vi "Create Sequence Call Step.vi"(8 "error in (no error)":errorcluster, 11 "QPA Measurement in":refnum<class "QPA Measurement.lvclass">) -> (0 "error out":errorcluster, 2 "Step Reference":refnum<k7>, 3 "QPA Measurement out":refnum<class "QPA Measurement.lvclass">)   [LabVIEW 2016, in "QPA Measurement.lvlib" / "QPA Measurement.lvclass"]
uses:
  QPA Measurement.lvclass
  C:/Projects/STS/Common/Sequence Automation/Plugins/Measurement Interface.lvlibp/Measurement Interface.lvclass
  QPA Measurement.lvclass/QPA Measurement.ctl
  Protected Methods/Read Sequence Reference.vi
  Protected Methods/Read Measurement Name.vi
  Plugins/Measurement Interface.lvlibp/Private Methods/Engine Reference/Read Engine Reference.vi
  Plugins/Measurement Interface.lvlibp/Private Methods/Measurement Parameters/Read Measurement Parameters.vi
  Plugins/String Database.lvlibp/String Database.lvclass
  Plugins/TestStand API Tools (TSAT).lvlibp/Step Actions/TSAT Step Actions.lvlib
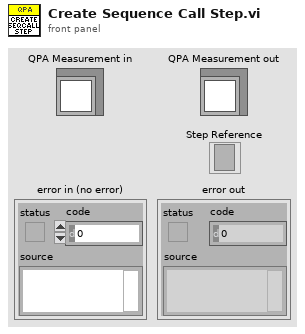
[diagram p1: front panel]
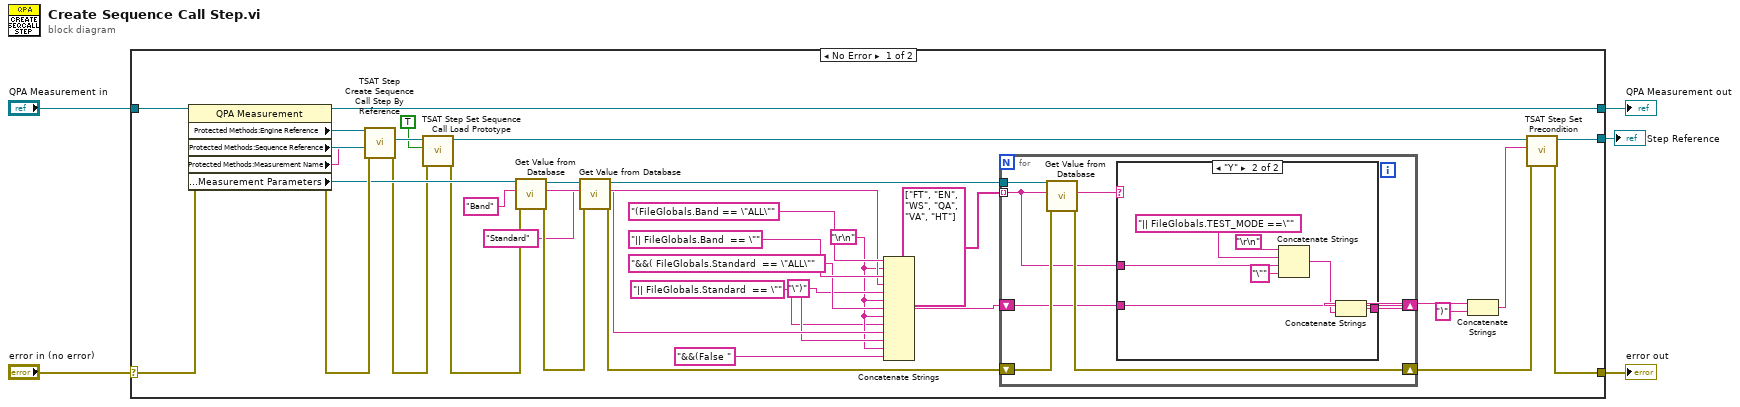
[diagram p0: block diagram]
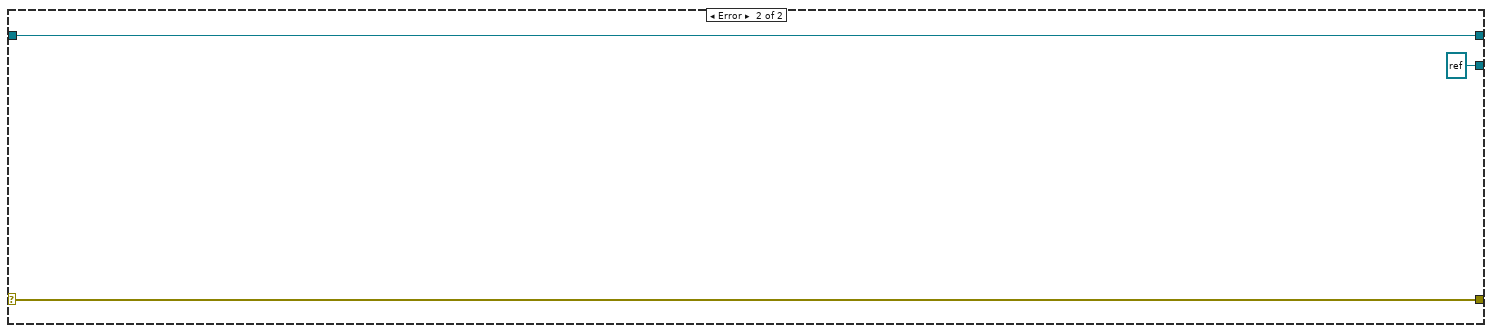
[diagram p3: hidden frame]
diagram:
  n1 = case shown="No Error" "error in (no error)" {
    selector: "error in (no error)" -> [w41 w59]
    tunnel: [w30 w59] -> w4
    tunnel: [w39 w58] -> w2
    tunnel: "QPA Measurement in" -> [w40 w58]
    tunnel: [w34 refnum<k7> refnum ("Step Reference")] -> w1
    frame No Error {
      w7 = "\r\n"
      w8 = "\")" ("string")
      n2 = property class="QPA Measurement"(reference=w40, error in=w41) -> (reference out=w39:refnum<class "QPA Measurement.lvclass">, error out=w35:errorcluster, "Protected Methods:Engine Reference"=w38:refnum<k7>, "Protected Methods:Sequence Reference"=w37:refnum<k7>, "Protected Methods:Measurement Name"=w36:string, "Protected Methods:Measurement Parameters"=w33:refnum<class "String Database.lvclass">)
      n3 = call "TSAT Step Create Sequence Call Step By Reference.vi"("Error In"=w35, "Step Name"=w36, "Sequence to Call"=w37, "Engine In"=w38) -> ("Error Out"=w31:errorcluster, "Step Reference"=w18:refnum<k7>)  [unwired: 5 in, 1 out]
      n4 = call "TSAT Step Set Sequence Call Load Prototype.vi"("Error In"=w31, "UseSequenceParameterPrototype"=TRUE, "Step In"=w18) -> ("Error Out"=w19:errorcluster, "Step Reference"=w17:refnum<k7>)  [unwired: 7 in]
      n5 = call "Get Value from Database.vi"("error in (no error)"=w19, "Entry Name"="Band", "Message in"=w33) -> ("error out"=w28:errorcluster, "Entry Value"=w20:string, "Message out"=w14:refnum<class "String Database.lvclass">)  [unwired: 5 in, 1 out]
      n6 = call "Get Value from Database.vi"("error in (no error)"=w28, "Entry Name"="Standard", "Message in"=w14) -> ("error out"=w15:errorcluster, "Entry Value"=w9:string, "Message out"=w13:refnum<class "String Database.lvclass">)  [unwired: 5 in, 1 out]
      n7 = Concatenate Strings("(FileGlobals.Band == \"ALL\"" ("string"), w7, "|| FileGlobals.Band  == \"", w20, w8, w7, "&&( FileGlobals.Standard  == \"ALL\"", w7, "|| FileGlobals.Standard  == \"", w9, w8, w7, "&&(False ") -> (w26:string)
      n8 = for {
        tunnel: w13 -> [w48]
        tunnel: string[] ["FT", "EN", "WS", "QA", "VA", "HT"] -> [w44] mode=indexing
        shift-right: [w46] -> w27
        shift-left: w15 -> [w47]
        shift-right: [w42] -> w25
        shift-left: w26 -> [w43]
        n9 = call "Get Value from Database.vi"("error in (no error)"=w47, "Entry Name"=w44, "Message in"=w48) -> ("error out"=w46:errorcluster, "Entry Value"=w45:string)  [unwired: 5 in, 2 out]
        n10 = case shown="\"Y\"" w45 {
          tunnel: w44 -> [_ w55]
          tunnel: w43 -> [w49 w53]
          tunnel: [w49 w51] -> w42
          frame "False", Default {
          }
          frame "Y" {
            n11 = Concatenate Strings("\r\n", "|| FileGlobals.TEST_MODE ==\"", w55, "\"" ("string")) -> (w52:string)
            n12 = Concatenate Strings(w53, w52) -> (w51:string)
          }
        }
      }
      n13 = Concatenate Strings(w25, ")" ("string")) -> (w23:string)
      n14 = call "TSAT Step Set Precondition.vi"("Error In"=w27, "Precondition"=w23, "Step In"=w17) -> ("Error Out"=w30:errorcluster, "Step Out"=w34:refnum<k7>)  [unwired: 7 in]
    }
    frame Error {
    }
  }
  "error out" <- w4
  "QPA Measurement out" <- w2
  "Step Reference" <- w1
